vi "Ejercicio 2.3.vi"() -> ()   [LabVIEW 2013]
panel:
  in  "Boolean":bool
  in  "stop 2":bool
  out "Waveform Graph":dbl[](graph)
  in  "Amplitud":dbl
  in  "Frecuencia":dbl
  in  "Cantidad de muestras":i32=20
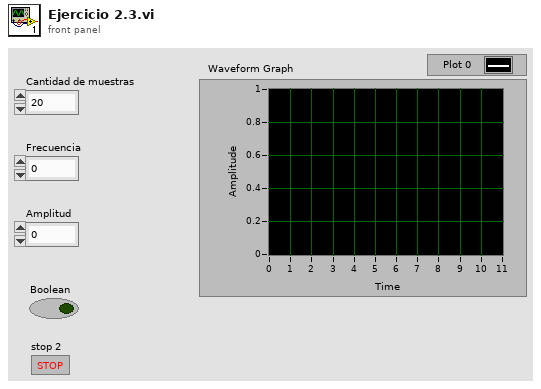
[diagram p1: front panel]
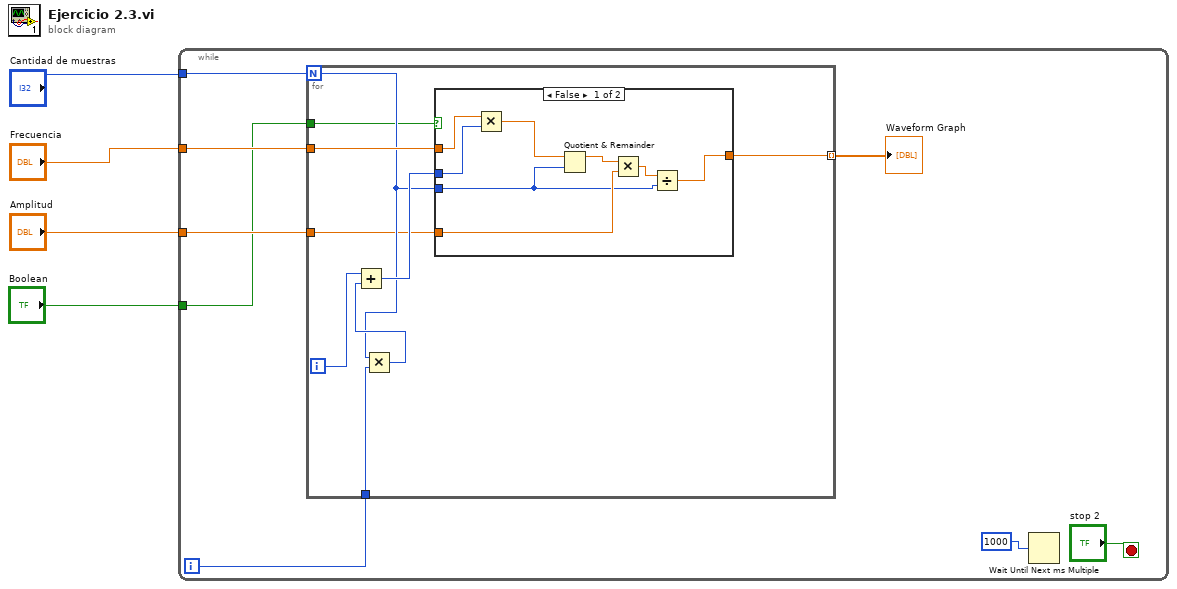
[diagram p0: block diagram]
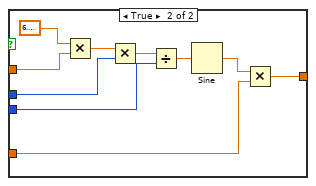
[diagram p2: hidden frame]
diagram:
  n1 = while {
    tunnel: "Cantidad de muestras" -> [w10]
    tunnel: "Frecuencia" -> [w7]
    tunnel: "Amplitud" -> [w9]
    tunnel: "Boolean" -> [w5]
    i -> [w8]
    stop <- "stop 2" stop-if-true
    n2 = for {
      N: w10 -> [w16]
      tunnel: w9 -> [w15]
      tunnel: w8 -> [w19]
      tunnel: w7 -> [w18]
      tunnel: [w14] -> w6 mode=indexing
      tunnel: w5 -> [w13]
      i -> [w21]
      n3 = Multiply(x=w16, y=w19) -> (x*y=w20:i32)
      n4 = Add(x=w21, y=w20) -> (x+y=w17:i32)
      n5 = case shown="False" w13 {
        tunnel: w18 -> [w29 w38]
        tunnel: w17 -> [w28 w36]
        tunnel: w16 -> [w23 w34]
        tunnel: w15 -> [w25 w31]
        tunnel: [w22 w30] -> w14
        frame False {
          n6 = Multiply(x=w29, y=w28) -> (x*y=w27:dbl)
          n7 = Quotient & Remainder(x=w27, y=w23) -> (x-y*floor(x/y)=w26:dbl)  [unwired: 1 out]
          n8 = Multiply(x=w26, y=w25) -> (x*y=w24:dbl)
          n9 = Divide(x=w24, y=w23) -> (x/y=w22:dbl)
        }
        frame True {
          n10 = Multiply(x=6.283185307179586, y=w38) -> (x*y=w37:dbl)
          n11 = Multiply(x=w37, y=w36) -> (x*y=w35:dbl)
          n12 = Divide(x=w35, y=w34) -> (x/y=w33:dbl)
          n13 = Sine(x=w33) -> (sin(x)=w32:dbl)
          n14 = Multiply(x=w32, y=w31) -> (x*y=w30:dbl)
        }
      }
    }
    "Waveform Graph" <- w6
    n15 = Wait Until Next ms Multiple(millisecond multiple=1000) -> ()  [unwired: 1 out]
  }
